vi "Generate SysDef Path.vi"() -> (0 "SysDef path":path)   [LabVIEW 2018, in "DMA Channels Interleaved Testing.lvclass"]
uses:
  DMA Channels Interleaved Testing.lvclass
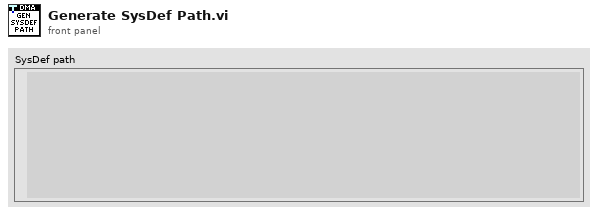
[diagram p1: front panel]
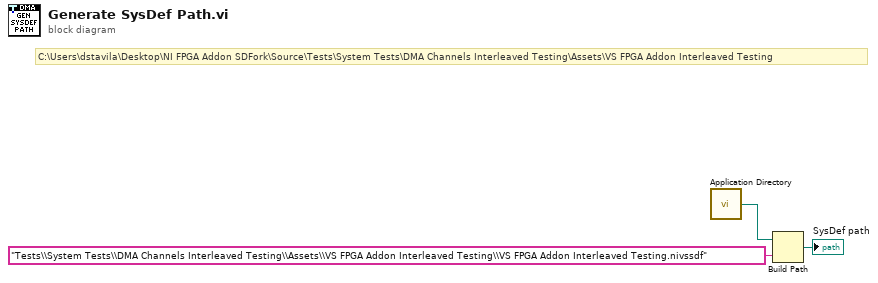
[diagram p0: block diagram]
diagram:
  # "C:\\Users\\dstavila\\Desktop\\NI FPGA Addon SDFork\\Source\\Tests\\System Tests\\DMA Channels Interleaved Testing\\Assets\\VS FPGA Addon Interleaved Testing"
  n1 = call <vilib>:"Application Directory.vi"() -> ("Application Directory"=w3:path)
  n2 = Build Path(base path=w3, name or relative path="Tests\\System Tests\\DMA Channels Interleaved Testing\\Assets\\VS FPGA Addon Interleaved Testing\\VS FPGA Addon Interleaved Testing.nivssdf") -> (appended path=→"SysDef path":path)
